vi "ActiveCMChannels.vi"(4 "CM_data":T1[](array[typedef])) -> (1 "ActiveChannels":i32)   [LabVIEW 2016]
uses:
  CurrentMeter/CM_data.ctl
  CurrentMeter/CM_SerialNumber.ctl
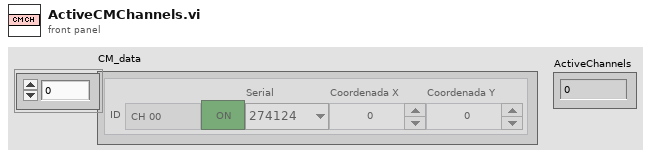
[diagram p1: front panel]
types:
  T1 = typedef "CM_data.ctl" = cluster{"Serial":T2, "Coordenada X":dbl, "Coordenada Y":dbl, "ID":string, "active":bool}
  T2 = typedef "CM_SerialNumber.ctl" = enum16{"274124", "274125", "274126", "274127", "274128"}
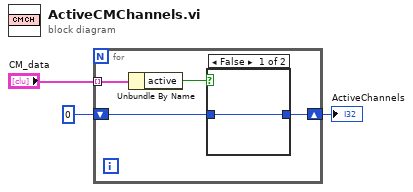
[diagram p0: block diagram]
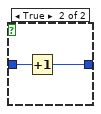
[diagram p2: hidden frame]
diagram:
  n1 = for {
    tunnel: "CM_data" -> [w7] mode=indexing
    shift-right: [w4] -> w3
    shift-left: 0 -> [w5]
    n2 = Unbundle By Name(w7) -> ("active"=w6:bool)
    n3 = case shown="False" w6 {
      tunnel: w5 -> [w8 w10]
      tunnel: [w8 w9] -> w4
      frame False {
      }
      frame True {
        n4 = Increment(x=w10) -> (x+1=w9:i32)
      }
    }
  }
  "ActiveChannels" <- w3
